vi "Slave RT Target.vi"() -> ()   [LabVIEW 2011]
uses:
  <vilib>/rvi/interface/nirviReadWriteControl/nirviReadWriteControl.xnode
  <vilib>/Utility/error.llb/Error Cluster From Error Code.vi
  <vilib>/rvi/errors/niLvFpgaAdjustHostInterfaceError.vi
  <vilib>/LabVIEW Targets/FPGA/cRIO/cRIO-9505/controls.llb/_nicrio_cRIO-9505_DriveStatus.ctl
  <vilib>/rvi/interface/nirviOpenFPGA/nirviOpenFPGA.xnode
  NiFpgaLv.dll
  <vilib>/rvi/interface/nirviCloseFPGA/nirviCloseFPGA.xnode
  FPGA/FPGA Bitfiles/SlaveInterface.lvbitx
  <vilib>/FPGAPlugInAG/cRIO-9114/niLvFpga_Open_cRIO-9114.vi
  <vilib>/FPGAPlugInAG/cRIO-9114/niLvFpga_Close_cRIO-9114.vi
panel:
  in  "Current PID Gains":T1={"Proportional Gain"=20, "Integral Gain"=5, "Derivative Gain"=0}
  in  "Current Limit (A)":dbl min=0.0 max=0.9 step=0.1
  out "Control Status":errorcluster
  in  "Control Rate (ms)":u32=1
  in  "Current Loop Rate (usec)":u32=50
  in  "Stop":bool
  in  "Read Port":u16=9090
  in  "UDP Rate (ms)":u32=1
  in  "Master IP":string="192.168.10.4"
  out "UDP Status":errorcluster
  in  "Write Port":u16=9595
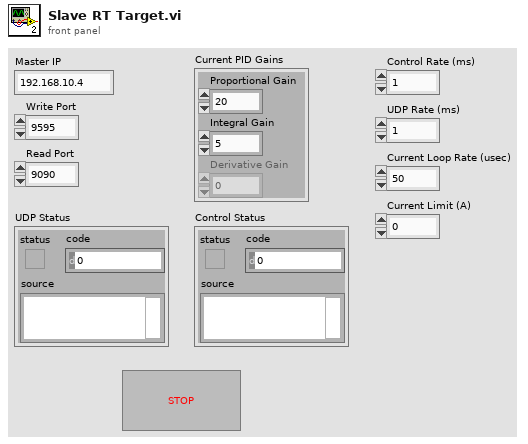
[diagram p1: front panel]
types:
  T1 = cluster{"Proportional Gain":i16, "Integral Gain":i16, "Derivative Gain":i16}
  T2 = typedef "_nicrio_cRIO-9505_DriveStatus.ctl" = enum8{"Enabled", "Disabled", "Disabled by Drive Fault", "Disabled by Temp. Fault", "Disabled by E-Stop", "Unknown"}
  T3 = enum16{"big-endian, network order", "native, host order", "little-endian"}
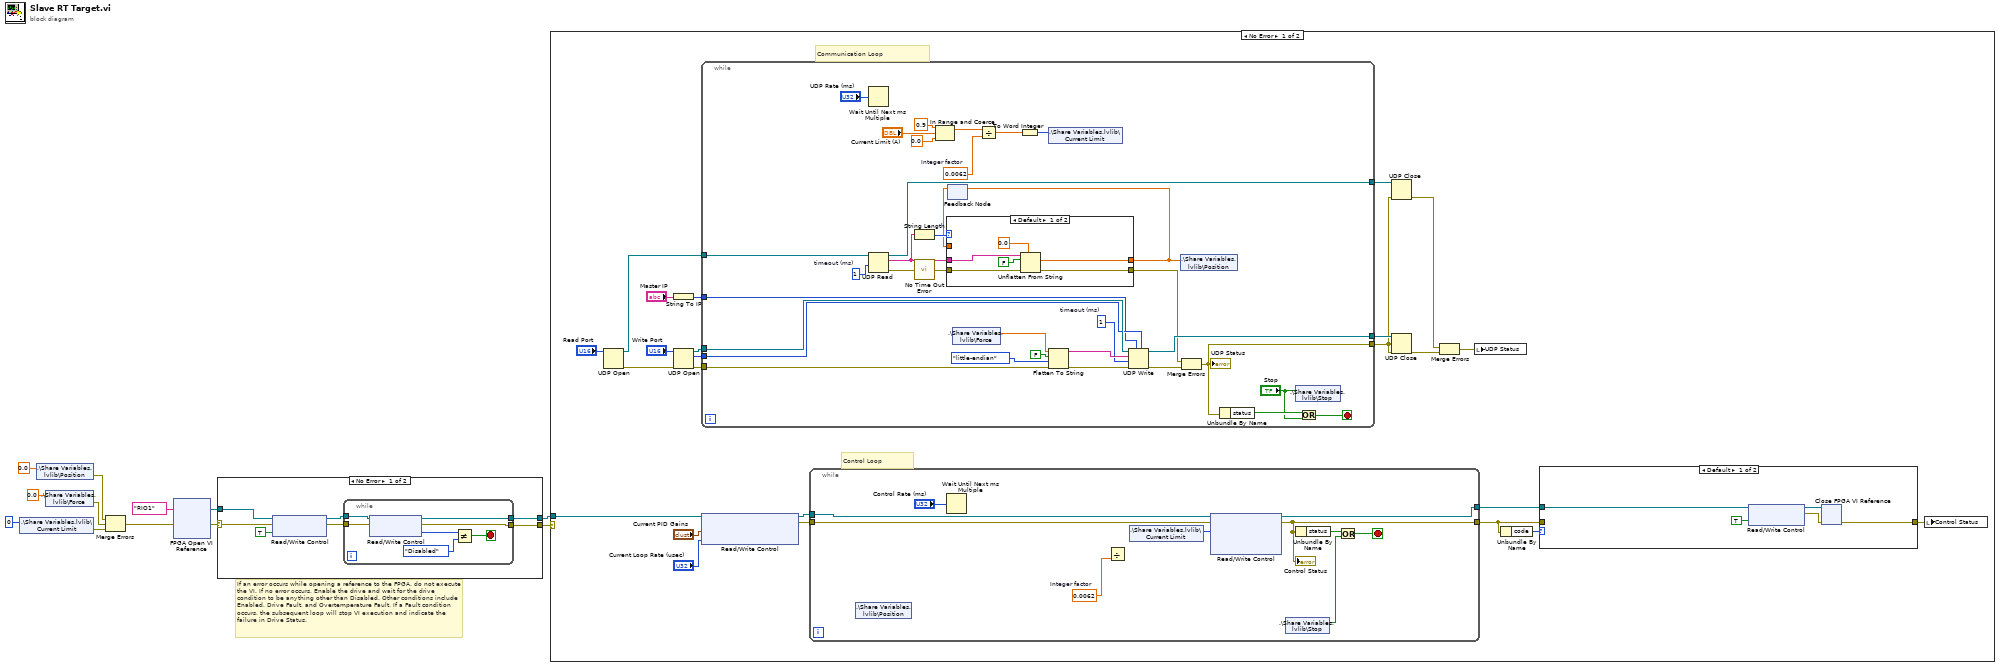
[diagram p0: block diagram]
diagram:
  # "If an error occurs while opening a reference to the FPGA, do not execute the VI. If no error occurs, Enable the drive and wait for the drive condition to be anything other than Disabled. Other conditions include Enabled, Drive Fault, and Overtemperature Fault. If a Fault condition occurs, the subsequent loop will stop VI execution and indicate the failure in Drive Status."
  n1 = shared-variable ".\\Share Variables.lvlib\\Current Limit"(i16 0 ("Current Limit")) -> (error out=w2:errorcluster)  [unwired: 1 in]
  n2 = shared-variable ".\\Share Variables.lvlib\\Position"(0.0 ("Position")) -> (error out=w7:errorcluster)  [unwired: 1 in]
  n3 = shared-variable ".\\Share Variables.lvlib\\Force"(0.0 ("Force")) -> (error out=w6:errorcluster)  [unwired: 1 in]
  n4 = Merge Errors(w7, w6, w2) -> (w5:errorcluster)
  n5 = xnode "FPGA Open VI Reference"("error in"=w5, "resource name"=tag "RIO1") -> ("FPGA VI Reference Out"=w12:refnum<k20>, "error out"=w11:errorcluster)
  n6 = case shown="No Error" w11 {
    selector: w11 -> [w14 w27]
    tunnel: w12 -> [w15 w28]
    tunnel: [w19 w28] -> w3
    tunnel: [w16 w27] -> w4
    frame No Error {
      n7 = xnode "Read/Write Control"("FPGA VI Reference In"=w15, "error in"=w14, "Enable Drive"=TRUE) -> ("FPGA VI Reference Out"=w18:refnum<k20>, "error out"=w17:errorcluster)
      n8 = while {
        tunnel: [w26] -> w19
        tunnel: w18 -> [w23]
        tunnel: w17 -> [w22]
        tunnel: [w24] -> w16
        stop <- w20 stop-if-true
        n9 = xnode "Read/Write Control"("FPGA VI Reference In"=w23, "error in"=w22) -> ("FPGA VI Reference Out"=w26:refnum<k20>, "error out"=w24:errorcluster, "Drive Status"=w21:T2)
        n10 = Not Equal?(x=w21, y=_nicrio_cRIO-9505_DriveStatus."Disabled") -> (x != y?=w20:bool)
      }
    }
    frame Error {
      # "Error occurred. Do not run."
    }
  }
  n11 = case shown="No Error" w4 {
    tunnel: w3 -> [w40 _]
    frame No Error {
      # "Control Loop"
      # "Communication Loop"
      n12 = UDP Open(11:"Read Port") -> (port=w45:refnum<k16>, 0:w44:errorcluster)  [unwired: 1 in, 4 out]
      n13 = String To IP(1:"Master IP") -> (0:w50:u32)
      n14 = UDP Open(8:w44, 11:"Write Port") -> (port=w49:refnum<k16>, 0:w43:errorcluster, 2:w48:u16)  [unwired: 3 out]
      n15 = while {
        tunnel: [w98] -> w47
        tunnel: w49 -> [w97]
        tunnel: w48 -> [w96]
        tunnel: w50 -> [w92]
        tunnel: w45 -> [w89]
        tunnel: [w85] -> w41
        tunnel: w43 -> [w87]
        tunnel: [w84] -> w42
        stop <- w91 stop-if-true
        w75 = 0.0062  # Integer factor
        w77 = 1  # timeout (ms)
        w100 = 1  # timeout (ms)
        n16 = Wait Until Next ms Multiple(millisecond multiple="UDP Rate (ms)") -> ()  [unwired: 1 out]
        n17 = UDP Read(connection ID=w89, timeout ms (25000)=w77) -> (data out=w83:string, error out=w90:errorcluster, 3:w84:refnum<k16>)  [unwired: 2 in, 2 out]
        n18 = String Length(string=w83) -> (length=w88:i32)
        n19 = call <vilib>:"No Time Out Error.vi"("error in (no error)"=w90) -> ("error out"=w82:errorcluster)  [unwired: 14 out]
        n20 = In Range and Coerce(upper limit=0.9 ("element"), x="Current Limit (A)", lower limit=0.0 ("element")) -> (coerced(x)=w69:dbl)  [unwired: 1 out]
        n21 = feedback #1() -> (w79:dbl)  [unwired: 1 in]
        n22 = case shown="Default" w88 {
          tunnel: w83 -> [w106 _]
          tunnel: w82 -> [w105 w110]
          tunnel: [w104 w110] -> w81
          tunnel: [w103 w109] -> w80
          tunnel: w79 -> [_ w109]
          frame Default {
            n23 = Unflatten From String(type=0.0, binary string=w106, data includes array or string size? (T)=FALSE, error in (no error)=w105) -> (value=w103:dbl, error out=w104:errorcluster)  [unwired: 2 out]
          }
          frame 0 {
          }
        }
        n24 = feedback-in #1(w80) -> ()
        n25 = shared-variable ".\\Share Variables.lvlib\\Force"() -> (w78:dbl)  [unwired: 1 in, 1 out]
        n26 = Divide(x=w69, y=w75) -> (x/y=w74:dbl)
        n27 = To Word Integer(number=w74) -> (16bit integer=w73:i16)
        n28 = shared-variable ".\\Share Variables.lvlib\\Current Limit"(w73) -> ()  [unwired: 1 in, 1 out]
        n29 = Flatten To String(anything=w78, prepend array or string size? (T)=FALSE, byte order (0:big-endian, network order)=T3."little-endian" ("Byte order"), error in (no error)=w87) -> (data string=w101:string, error out=w99:errorcluster)  [unwired: 1 out]
        n30 = UDP Write(address=w92, port or service name=w96, connection ID=w97, data in=w101, 8:w99, 9:w100) -> (error out=w86:errorcluster, 3:w98:refnum<k16>)
        n31 = shared-variable ".\\Share Variables.lvlib\\Position"(w80) -> ()  [unwired: 1 in, 1 out]
        n32 = Merge Errors(w81, w86) -> (w85:errorcluster)
        "UDP Status" <- w85
        n33 = Unbundle By Name(w85) -> ("status"=w95:bool)
        n34 = shared-variable ".\\Share Variables.lvlib\\Stop"("Stop") -> ()  [unwired: 1 in, 1 out]
        n35 = Or(x=w95, y="Stop") -> (x .or. y?=w91:bool)
      }
      n36 = xnode "Read/Write Control"("FPGA VI Reference In"=w40, "Current PI Gains"="Current PID Gains", "Current Loop Rate (usec)"="Current Loop Rate (usec)") -> ("FPGA VI Reference Out"=w39:refnum<k20>, "error out"=w38:errorcluster)  [unwired: 1 in]
      n37 = while {
        tunnel: w39 -> [w68]
        tunnel: w38 -> [w67]
        tunnel: [w65] -> w35
        tunnel: [w60] -> w34
        stop <- w61 stop-if-true
        w59 = 0.0062  # Integer factor
        n38 = shared-variable ".\\Share Variables.lvlib\\Position"() -> ()  [unwired: 1 in, 2 out]
        n39 = Wait Until Next ms Multiple(millisecond multiple="Control Rate (ms)") -> ()  [unwired: 1 out]
        n40 = Divide(y=w59) -> ()  [unwired: 1 in, 1 out]
        n41 = shared-variable ".\\Share Variables.lvlib\\Current Limit"() -> (w66:i16)  [unwired: 1 in, 1 out]
        n42 = xnode "Read/Write Control"("FPGA VI Reference In"=w68, "error in"=w67, "Current Limit"=w66) -> ("FPGA VI Reference Out"=w65:refnum<k20>, "error out"=w60:errorcluster)  [unwired: 1 in, 1 out]
        "Control Status" <- w60
        n43 = shared-variable ".\\Share Variables.lvlib\\Stop"() -> (w63:bool)  [unwired: 1 in, 1 out]
        n44 = Unbundle By Name(w60) -> ("status"=w62:bool)
        n45 = Or(x=w62, y=w63) -> (x .or. y?=w61:bool)
      }
      n46 = UDP Close(connection ID=w42, 8:w41) -> (error out=w32:errorcluster)  [unwired: 1 out]
      n47 = UDP Close(connection ID=w47, 8:w41) -> (error out=w31:errorcluster)  [unwired: 1 out]
      n48 = Merge Errors(w32, w31) -> (w30:errorcluster)
      n49 = local write "UDP Status"(w30) -> ()
      n50 = Unbundle By Name(w34) -> ("code"=w36:i32)
      n51 = case shown="Default" w36 {
        tunnel: [w55 w58] -> w33
        tunnel: w35 -> [w54 _]
        tunnel: w34 -> [_ w58]
        frame Default {
          n52 = xnode "Read/Write Control"("FPGA VI Reference In"=w54, "Disable Drive"=TRUE ("Disable Motors")) -> ("FPGA VI Reference Out"=w57:refnum<k20>, "error out"=w56:errorcluster)  [unwired: 1 in]
          n53 = xnode "Close FPGA VI Reference"("FPGA VI Reference In"=w57, "error in"=w56) -> ("error out"=w55:errorcluster)
        }
        frame -65536 {
          # "Unable to communicate with the module. Reinsert the module and check connections.\nIf the chassis is in FPGA Interface programming mode, make sure you have opened an \nFPGA reference to a bitfile or FPGA VI with Scan Interface support for the module you are \ntrying to access using the Scan Interface."
        }
      }
      n54 = local write "Control Status"(w33) -> ()
    }
    frame Error {
    }
  }
